vi "DDS Pulse IO Update.vi"(7 "port number (0)":u8, 8 "error in (no error)":errorcluster, 10 "channel number (1)":u8=1 min=1 max=4 step=1, 11 "spi script reference in":T1) -> (0 "error out":errorcluster, 3 "spi script reference out":T1)   [LabVIEW 2013, in "DDS.lvlib"]
doc: "Pulses IO Update for the given channel (1 through 4 only)."
uses:
  DDS.lvlib
  <vilib>/ni845x/ni845x.llb/ni845xSpiScriptControl.ctl
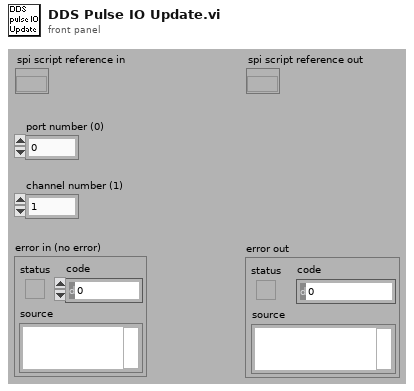
[diagram p1: front panel]
types:
  T1 = typedef "ni845xSpiScriptControl.ctl" = refnum<k20>
  T2 = typedef "DDS.lvlib/DDS DIO pins.ctl" = enum8{"Ch. 4 master reset", "Ch. 3 master reset", "Ch. 2 master reset", "Ch. 1 master reset", "Ch. 1 IO update", "Ch. 2 IO update", "Ch. 3 IO update", "Ch. 4 IO update"}
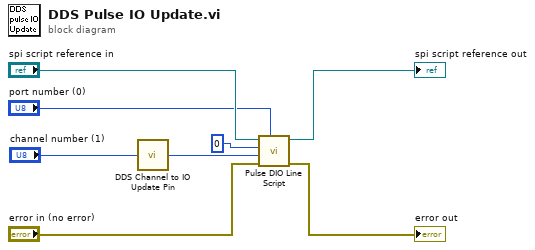
[diagram p0: block diagram]
diagram:
  n1 = call "DDS Channel to IO Update Pin.vi"("channel number (1)"="channel number (1)") -> ("DIO pin"=w2:T2)
  n2 = call "Pulse DIO Line Script.vi"("port number (0)"="port number (0)", "error in (no error)"="error in (no error)", "DIO line number (0)"=w2, "pulse width delay [ms] (0)"=u8 0, "spi script reference in"="spi script reference in") -> ("error out"=→"error out":errorcluster, "spi script reference out"=→"spi script reference out":T1)  [unwired: 5 in]
